vi "setDeviceParameters.vi"(8 "error in (no error)":errorcluster, 11 "cRIO in":refnum<class "cRIO.lvclass">) -> (0 "error out":errorcluster, 3 "cRIO out":refnum<class "cRIO.lvclass">)   [LabVIEW 2020, in "cRIO.lvclass"]
uses:
  cRIO.lvclass
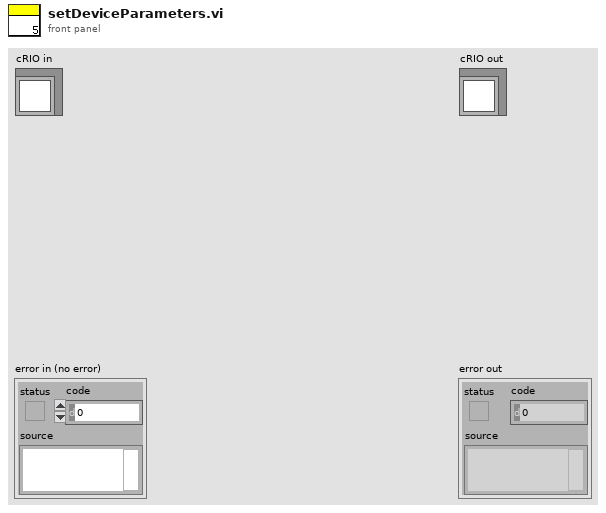
[diagram p1: front panel]
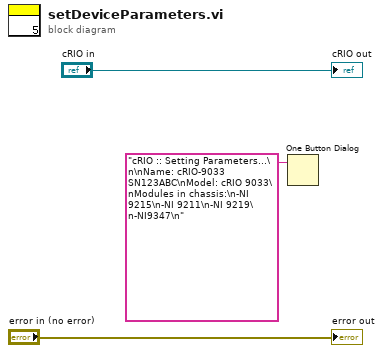
[diagram p0: block diagram]
diagram:
  n1 = One Button Dialog(message="cRIO :: Setting Parameters...\n\nName: cRIO-9033 SN123ABC\nModel: cRIO 9033\nModules in chassis:\n-NI 9215\n-NI 9211\n-NI 9219\n-NI9347\n") -> ()  [unwired: 1 in, 1 out]
  "error out" <- "error in (no error)"
  "cRIO out" <- "cRIO in"
